vi "modify.vi"(1 "consequence":T1(array[cluster])=[{"ling.var."="out", "x-min"=-1.0, "x-max"=1.0, "setarray"=[{"linguistic term"="NEo", "color"=16711680, "points"=[-1.0, -1.0, -1.0, 0.0]}, {"linguistic term"="ZEo", "color"=255, "points"=[-1.0, 0.0, 0.0, 1.0]}, {"linguistic term"="POo", "color"=26214, "points"=[0.0, 1.0, 1.0, 1.0]}]}] {"x-min" format="%.2f"; "x-max" format="%.2f"; "setarray"."points" min=-1.0 max=1.0 step=0.10000000149011612 format="%.2f"}) -> (0 "consequence modified":T1(array[cluster])=[{"ling.var."="out", "x-min"=-2.0, "x-max"=2.0, "setarray"=[{"linguistic term"="NEo", "color"=16711680, "points"=[-2.0, -1.0, -1.0, 0.0]}, {"linguistic term"="ZEo", "color"=255, "points"=[-1.0, 0.0, 0.0, 1.0]}, {"linguistic term"="POo", "color"=26214, "points"=[0.0, 1.0, 1.0, 2.0]}]}] {"x-min" format="%.2f"; "x-max" format="%.2f"; "setarray"."points" min=-1.0 max=1.0 step=0.10000000149011612 format="%.2f"})   [LabVIEW 2020, in "NI_fuzzy logic.lvlib"]
doc: "This VI modifies the consequenceterms. \nSets at the range limitation are mirrored and the range is spreaded.\nIt«s needed to use the complete range adjustment of the controlleroutput."
uses:
  <vilib>/addons/control/fuzzy/NI_fuzzy logic.lvlib
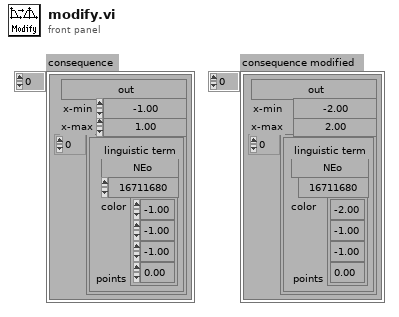
[diagram p1: front panel]
types:
  T1 = cluster{"ling.var.":string, "x-min":dbl, "x-max":dbl, "setarray":cluster{"linguistic term":string, "color":u32, "points":dbl[]}[]}[]
  T2 = cluster{"linguistic term":string, "color":u32, "points":dbl[]}[]
  T3 = cluster{"points[0]":dbl, "points[1]":dbl, "points[2]":dbl, "points[3]":dbl}
  T4 = cluster{"linguistic term":string, "color":u32, "points":dbl[]}
  T5 = cluster{"ling.var.":string, "x-min":dbl, "x-max":dbl, "setarray":cluster{"linguistic term":string, "color":u32, "points":dbl[]}[]}
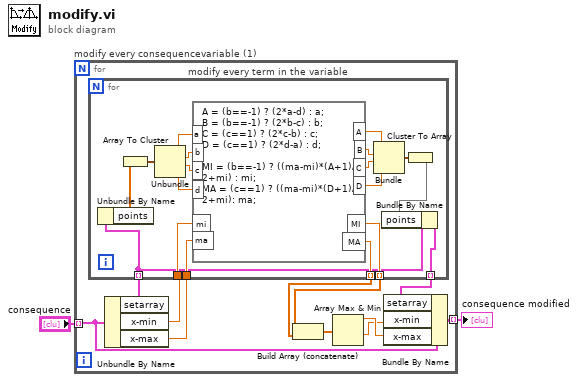
[diagram p0: block diagram]
diagram:
  n1 = for "modify every consequencevariable (1)" {
    tunnel: "consequence" -> [w3] mode=indexing
    tunnel: [w9] -> w1 mode=indexing
    n2 = Unbundle By Name(w3) -> ("setarray"=w13:T2, "x-min"=w12:dbl, "x-max"=w11:dbl)
    n3 = for "modify every term in the variable" {
      tunnel: w13 -> [w14] mode=indexing
      tunnel: w12 -> [w20]
      tunnel: w11 -> [w19]
      tunnel: [w18] -> w8 mode=indexing
      tunnel: [w15] -> w10 mode=indexing
      tunnel: [w17] -> w7 mode=indexing
      n4 = Unbundle By Name(w14) -> ("points"=w21:dbl[])
      n5 = Array To Cluster(array=w21) -> (cluster=w30:T3)
      n6 = Unbundle(w30) -> ("points[0]"=w29:dbl, "points[1]"=w28:dbl, "points[2]"=w27:dbl, "points[3]"=w31:dbl)
      n7 = formula code="A = (b==-1) ? (2*a-d) : a;\nB = (b==-1) ? (2*b-c) : b;\nC = (c==1) ? (2*c-b) : c;\nD = (c==1) ? (2*d-a) : d;\n\nMI = (b==-1) ? ((ma-mi)*(A+1)/2+mi) : mi;\nMA = (c==1) ? ((ma-mi)*(D+1)/2+mi): ma;"("a"=w29, "b"=w28, "c"=w27, "d"=w31, "mi"=w20, "ma"=w19) -> ("A"=w26:dbl, "B"=w23:dbl, "C"=w24:dbl, "D"=w25:dbl, "MI"=w17:dbl, "MA"=w18:dbl)
      n8 = Bundle("A"=w26, "B"=w23, "C"=w24, "D"=w25) -> (w22:cluster{"A":dbl, "B":dbl, "C":dbl, "D":dbl})  [unwired: 1 out]
      n9 = Cluster To Array(cluster=w22) -> (array=w16:dbl[])
      n10 = Bundle By Name(cluster=w14, "points"=w16) -> (w15:T4)
    }
    n11 = Build Array (concatenate)(w7, w8) -> (w6:dbl[])
    n12 = Array Max & Min(array=w6) -> (max value=w5:dbl, min value=w4:dbl)  [unwired: 2 out]
    n13 = Bundle By Name(cluster=w3, "setarray"=w10, "x-min"=w4, "x-max"=w5) -> (w9:T5)
  }
  "consequence modified" <- w1
